vi "CmdSetAttenuatorEnable.vi"(8 "error in (no error)":errorcluster, 9 "Attenuator Enable":i32, 10 "Device Key In":string, 11 "CmdLib In":refnum<k24>) -> (0 "error out":errorcluster, 1 "IOStatus":i32, 2 "Device Key Out":string, 3 "CmdLib Out":refnum<k24>)   [LabVIEW 2010]
uses:
  C:/Code/Apps/Utilities/PM2935/PMWinApp/PM_Installer/Master/Samples/1918 - 2936 Family/LabVIEW/LabVIEW 2010/PowerMeterCommands.dll
  PowerMeterCommands.dll
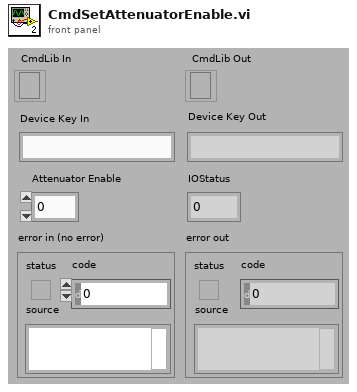
[diagram p1: front panel]
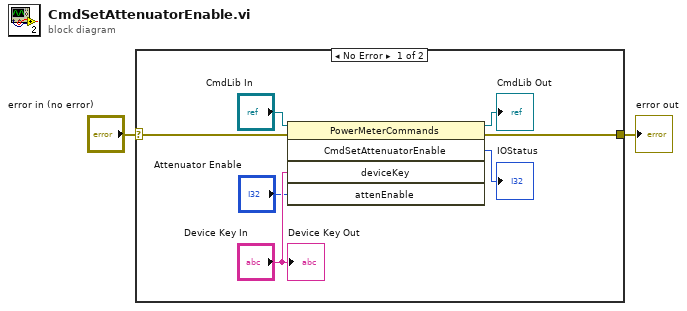
[diagram p0: block diagram]
diagram:
  n1 = case shown="No Error" "error in (no error)" {
    selector: "error in (no error)" -> [w5 w10]
    tunnel: [w4 w10] -> w1
    frame No Error {
      n2 = invoke class="PowerMeterCommands" method="CmdSetAttenuatorEnable"(reference="CmdLib In", error in=w5, "deviceKey"="Device Key In", "attenEnable"="Attenuator Enable") -> (reference out=→"CmdLib Out":refnum<k24>, error out=w4:errorcluster, "CmdSetAttenuatorEnable"=→"IOStatus":i32)  [unwired: 1 in, 2 out]
      "Device Key Out" <- "Device Key In"
    }
    frame Error {
    }
  }
  "error out" <- w1
